vi "WDTreset.vi"(6 "String":string) -> (0 "error out 2":errorcluster, 2 "String 2":string)   [LabVIEW 2010]
doc: "Перезапуск WDT"
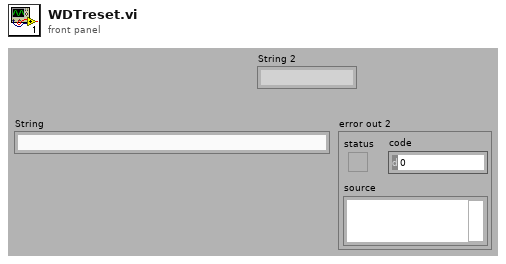
[diagram p1: front panel]
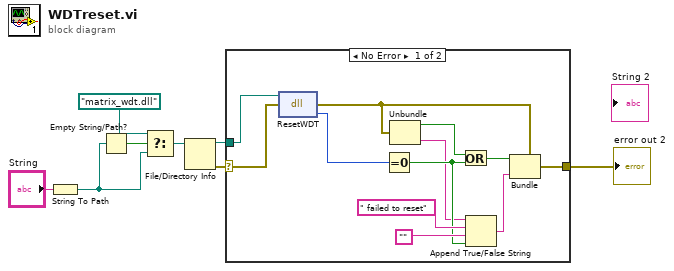
[diagram p0: block diagram]
diagram:
  n1 = String To Path(string="String") -> (path=w8:path)
  n2 = Empty String/Path?(string/path=w8) -> (empty?=w5:bool)
  n3 = Select(t=path "matrix_wdt.dll" ("WDTpath"), s=w5, f=w8) -> (s? t:f=w3:path)
  n4 = File/Directory Info(path=w3) -> (path out=w1:path, error out=w2:errorcluster)  [unwired: 1 in, 5 out]
  n5 = case shown="No Error" w2 {
    selector: w2 -> [w9 w21]
    tunnel: [w11 w21] -> w4
    tunnel: w1 -> [w10 _]
    frame No Error {
      n6 = dll-call lib="C:/AdLink/Matrix-4000/Lib/matrix_wdt.dll" fn="ResetWDT"(path in=w10, error in=w9) -> (error out=w20:errorcluster, "rezult"=w19:i32)  [unwired: 1 in, 1 out]
      n7 = Equal To 0?(x=w19) -> (x = 0?=w15:bool)
      n8 = Unbundle(w20) -> ("status"=w12:bool, "source"=w14:string)  [unwired: 1 out]
      n9 = Or(x=w12, y=w15) -> (x .or. y?=w13:bool)
      n10 = Append True/False String(1:w15, 2:"", 3:" failed to reset" ("true string"), 4:w14) -> (0:w16:string)
      n11 = Bundle(cluster=w20, "status"=w13, "source"=w16) -> (w11:errorcluster)  [unwired: 1 in]
    }
    frame Error {
    }
  }
  "error out 2" <- w4
